vi "celsius_to_fahrenhite.vi"() -> ()   [LabVIEW 2019]
panel:
  out "Fahrenheit":dbl
  in  "Celsius":dbl
  # "Convertion of temperature from\n         celsius to fahrenheit"
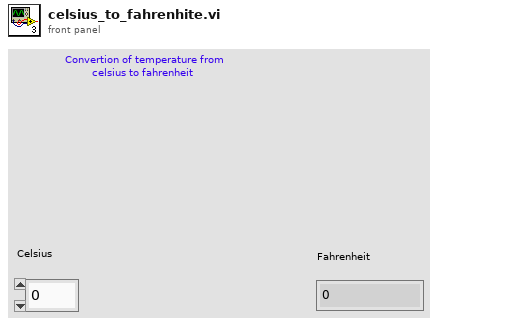
[diagram p1: front panel]
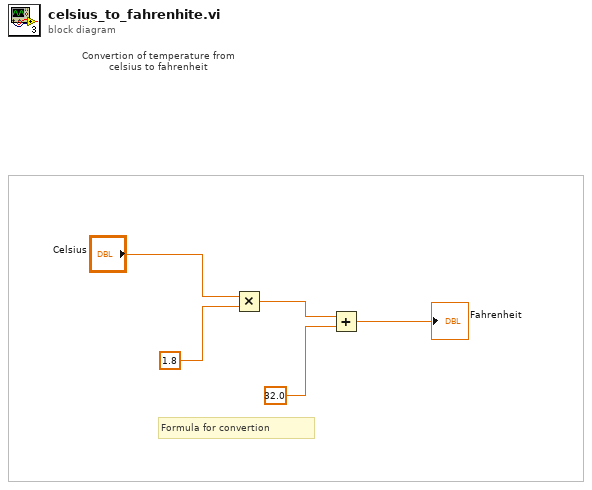
[diagram p0: block diagram]
diagram:
  # "Formula for convertion"
  # "Convertion of temperature from\n         celsius to fahrenheit"
  n1 = Multiply(x="Celsius", y=1.8) -> (x*y=w3:dbl)
  n2 = Add(x=w3, y=32.0) -> (x+y=→"Fahrenheit":dbl)
